vi "example_llm_openai_unit_test_1.vi"() -> ()   [LabVIEW 2020]
uses:
  src/models/llm_openai_chatmodels/llm_openai_chatmodels.lvclass
  D:/petwork/labview-llm-libraries-review/src/models/abstract_llm_base/abstract_llm_base.lvclass
  src/models/message_text/message_text.lvclass
  D:/petwork/labview-llm-libraries-review/src/models/abstract_message_base/abstract_message_base.lvclass
  src/models/message_text/message.ctl
panel:
  in  "temperature":dbl=1.0
  in  "Messages":cluster{"role":string, "text":string}[](array[cluster])=[{"role"="system", "text"="Act as a math teacher and guide the student in solving the problem. You should not solve the problem. Always answer in single line."}, {"role"="user", "text"="What is x in the equation 2x + 3 = 5  ?"}]
  out "error out":errorcluster
  out "openai_key":string
  in  "model_name":string(combo)="gpt-4o-mini"
  # "1. Ensure you assign the OpenAI Key to environmental variables so it is away from the code and easy to use the examples in future.\n\n2. Use the \"Set_ENv_Var.vi\" from examples/utils folder to set the key \"labview_llm_openai_key\"."
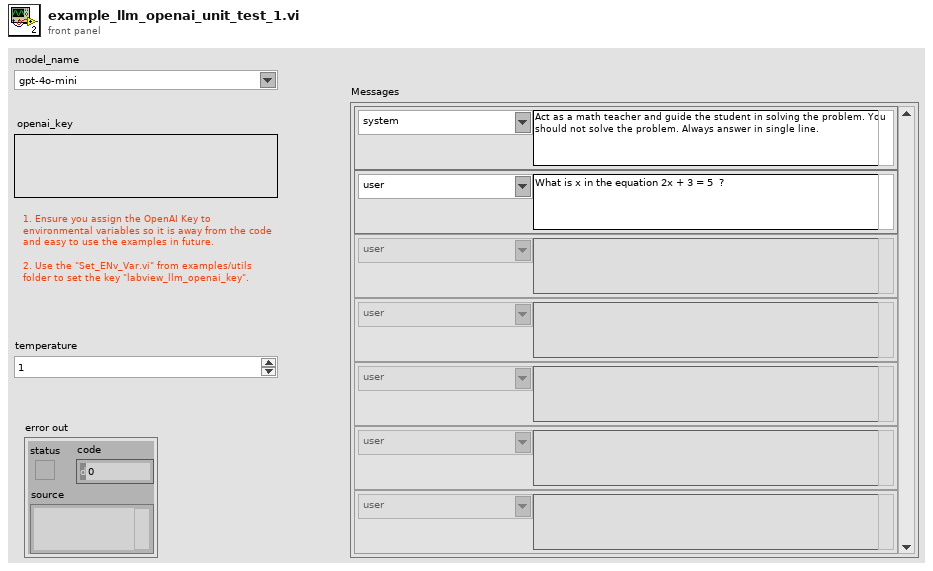
[diagram p1: front panel]
types:
  T1 = typedef "message_text.lvclass/message.ctl" = cluster{"role":string, "content":string[]}
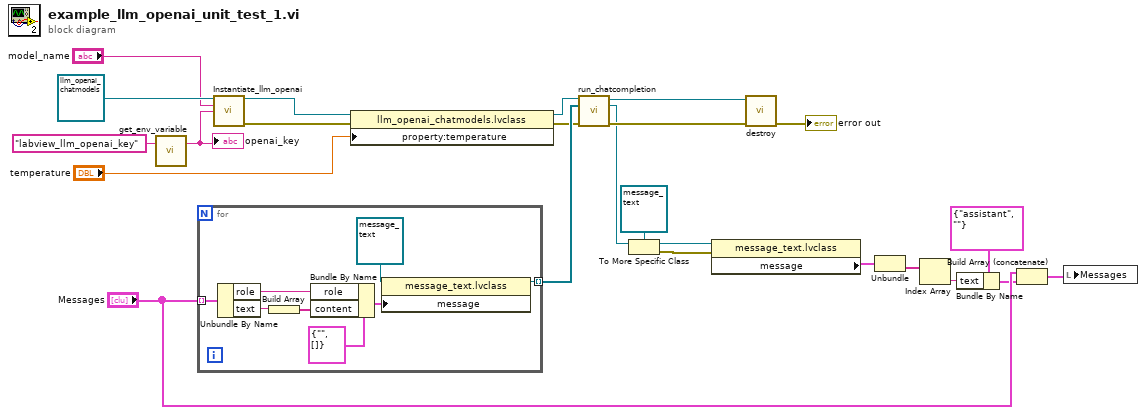
[diagram p0: block diagram]
diagram:
  n1 = call "get_env_variable.vi"("Environment Variable Name"="labview_llm_openai_key") -> ("Value"=w19:string)  [unwired: 1 in, 1 out]
  "openai_key" <- w19
  n2 = for {
    tunnel: "Messages" -> [w30] mode=indexing
    tunnel: [w31] -> w16 mode=indexing
    n3 = Unbundle By Name(w30) -> ("role"=w28:string, "text"=w26:string)
    n4 = Build Array(w26) -> (w25:string[])
    n5 = Bundle By Name(cluster=T1 {"role"="", "content"=[]} ("message"), "role"=w28, "content"=w25) -> (w27:T1)
    n6 = property class="message_text.lvclass"(reference=refnum<class "message_text.lvclass"> refnum ("message_text.lvclass"), "message"=w27) -> (reference out=w31:refnum<class "message_text.lvclass">)  [unwired: 1 in, 1 out]
  }
  n7 = call "Instantiate_llm_openai.vi"("llm_openai in"=refnum<class "llm_openai_chatmodels.lvclass"> refnum, "model_name"="model_name", "openai_key"=w19) -> ("llm_openai out"=w24:refnum<class "llm_openai_chatmodels.lvclass">, "error out"=w12:errorcluster)  [unwired: 11 in]
  n8 = property class="llm_openai_chatmodels.lvclass"(reference=w24, error in=w12, "property:temperature"="temperature") -> (reference out=w13:refnum<class "llm_openai_chatmodels.lvclass">, error out=w11:errorcluster)
  n9 = call-dynamic "run_chatcompletion.vi"("chatcompletion_llm_interface in"=w13, "Messages"=w16, "error in (no error)"=w11) -> ("chatcompletion_llm_interface out"=w21:refnum<class "llm_openai_chatmodels.lvclass">, "Response"=w2:refnum<class "abstract_message_base.lvclass">, "error out"=w20:errorcluster)  [unwired: 10 in]
  n10 = To More Specific Class(target class=refnum<class "message_text.lvclass"> refnum ("message_text.lvclass"), reference=w2) -> (specific class reference=w3:refnum<class "message_text.lvclass">, error out=w5:errorcluster)  [unwired: 1 in]
  n11 = property class="message_text.lvclass"(reference=w3, error in=w5) -> ("message"=w8:T1)  [unwired: 2 out]
  n12 = call-dynamic "destroy.vi"("error in (no error)"=w20, "abstract_llm_base in"=w21) -> ("error out"=→"error out":errorcluster)  [unwired: 8 in, 1 out]
  n13 = Unbundle(w8) -> ("content"=w7:string[])  [unwired: 1 out]
  n14 = Index Array(array=w7) -> (element=w6:string)  [unwired: 1 in]
  n15 = Bundle By Name(cluster=cluster{"role":string, "text":string} {"role"="assistant", "text"=""} ("message"), "text"=w6) -> (w1:cluster{"role":string, "text":string})
  n16 = Build Array (concatenate)("Messages", w1) -> (w14:cluster{"role":string, "text":string}[])
  n17 = local write "Messages"(w14) -> ()
